vi "Test Incomplete Coverage Running Same Code Twice.vi"(8 "error in (no error)":errorcluster, 11 "Test Case In":refnum<class "Coverage Test.lvclass">) -> (0 "error out":errorcluster, 3 "Test Case Out":refnum<class "Coverage Test.lvclass">)   [LabVIEW 2020, in "LUnit Tests.lvlib" / "Coverage Test.lvclass"]
uses:
  Coverage Test.lvclass
  C:/Program Files (x86)/National Instruments/LabVIEW 2020/vi.lib/Astemes/LUnit/Test Case.lvclass
  source/Framework/Coverage Analyzer/Coverage Analyzer.lvclass
  <vilib>/Astemes/LUnit/Test Case.lvclass/Test Case.ctl
  <vilib>/Astemes/LUnit/LUnit Assertion Result.lvclass/LUnit Assertion Result.ctl
  <vilib>/Astemes/LUnit/LUnit Test Case Result.lvclass/LUnit Test Case Result.ctl
  <vilib>/Astemes/LUnit/LUnit Method Result.lvclass/LUnit Method Result.ctl
  e50610f8-1631-4f30-8333-0e7769afa022.vi
  <vilib>/Astemes/LUnit/Set Assertion Type.vi
  <vilib>/Astemes/LUnit/Palette/Pass.vi
  <vilib>/Astemes/LUnit/Palette/Fail.vi
  <vilib>/Astemes/LUnit/Compare Variants.vi
  <vilib>/Astemes/LUnit/Describe Comparison.vi
  <vilib>/Astemes/LUnit/LUnit Write Assertion Type.vi
  <vilib>/Astemes/LUnit/Add test result.vi
  <vilib>/Astemes/LUnit/LUnit Write Passed.vi
  <vilib>/Astemes/LUnit/LUnit Write Message.vi
  <vilib>/Astemes/LUnit/LUnit Write Description.vi
  <vilib>/Astemes/LUnit/Variant to string.vi
  <vilib>/Astemes/LUnit/LUnit Record Assertion Result.vi
  <vilib>/Astemes/LUnit/LUnit Aggregate Assertion Results.vi
  <vilib>/Astemes/LUnit/Assertion Result/LUnit Read Status.vi
  <vilib>/Astemes/LUnit/LUnit Read Message.vi
  <vilib>/Astemes/LUnit/LUnit Read Description.vi
  <vilib>/Astemes/LUnit/Method Result/LUnit Merge Status.vi
  <vilib>/Astemes/LUnit/LUnit Concatenate result strings.vi
  <vilib>/Utility/Data Type/Get Type Information.vi
  <vilib>/Utility/LVClass/Get LV Class Name.vi
  <vilib>/Astemes/LUnit/LUnit Assertion Result.lvclass
  <vilib>/Astemes/LUnit/Test Case.lvclass
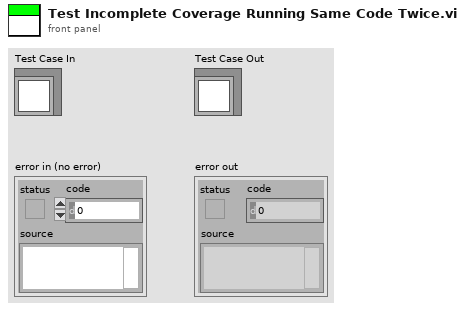
[diagram p1: front panel]
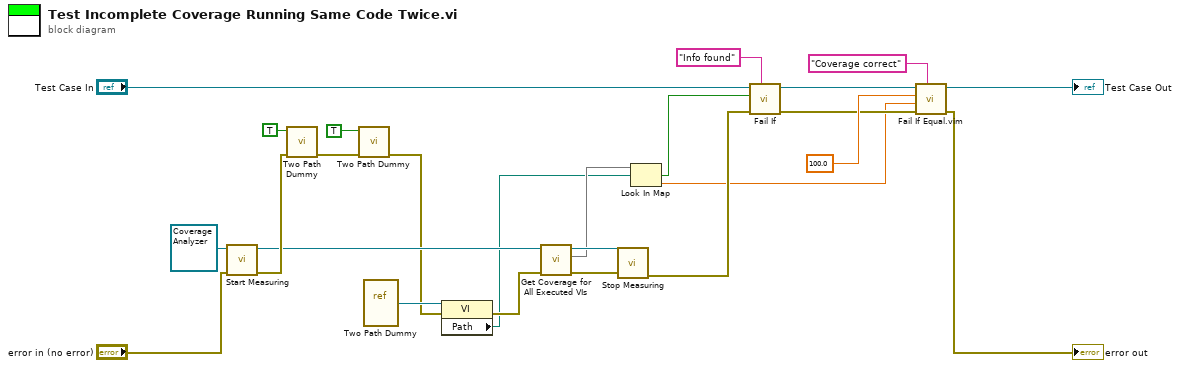
[diagram p0: block diagram]
diagram:
  n1 = call "Start Measuring.vi"("error in (no error)"="error in (no error)", "Coverage Analyzer in"=refnum<class "Coverage Analyzer.lvclass"> refnum) -> ("error out"=w16:errorcluster, "Coverage Analyzer out"=w15:refnum<class "Coverage Analyzer.lvclass">)  [unwired: 8 in]
  n2 = call "Two Path Dummy.vi"("error in (no error)"=w16, "Boolean"=TRUE) -> ("error out"=w20:errorcluster)  [unwired: 9 in]
  n3 = call "Two Path Dummy.vi"("error in (no error)"=w20, "Boolean"=TRUE) -> ("error out"=w5:errorcluster)  [unwired: 9 in]
  n4 = vi-ref "Two Path Dummy.vi"() -> (w23:refnum<vi>)
  n5 = property class="VI"(reference=w23, error in=w5) -> (error out=w6:errorcluster, "Path"=w2:path)  [unwired: 1 out]
  n6 = call "Get Coverage for All Executed VIs.vi"("error in (no error)"=w6, "Coverage Analyzer in"=w15) -> ("error out"=w13:errorcluster, "Code Coverage"=w3:map{path, dbl}, "Coverage Analyzer out"=w14:refnum<class "Coverage Analyzer.lvclass">)  [unwired: 7 in]
  n7 = call "Stop Measuring.vi"("error in (no error)"=w13, "Coverage Analyzer in"=w14) -> ("error out"=w9:errorcluster)  [unwired: 8 in, 1 out]
  n8 = Look In Map(map=w3, key=w2) -> (key not found?=w1:bool, value=w4:dbl)  [unwired: 1 in]
  n9 = call <vilib>:"Fail If.vi"("Description"="Info found", "error in (no error)"=w9, "Fail?"=w1, "LUnit Test Case In"="Test Case In") -> ("error out"=w12:errorcluster, "LUnit Test Case Out"=w10:refnum<class "Coverage Test.lvclass">)  [unwired: 6 in]
  n10 = call "Fail If Equal.vim"("Description"="Coverage correct", "error in (no error)"=w12, "Actual"=w4, "Expected"=100.0 ("Coverage Percentage"), "LUnit Test Case In"=w10) -> ("error out"=→"error out":errorcluster, "LUnit Test Case Out"=→"Test Case Out":refnum<class "Coverage Test.lvclass">)  [unwired: 5 in]
